vi "magTerm.vi"() -> ()   [LabVIEW 2014]
uses:
  common/crest/LabVIEW/LV14/libcommon-crest.lvlib
panel:
  out "loop":i32
  in  "Simulated/Real":string(combo)
  in  "stop":bool
  out "Array":T1(array[cluster])
  in  "!CHAOS WAN url":string="192.168.150.91:8081"
  in  "Element List":string[](array[string])=["DHSTB001", "DHSTB002", "QUATB001", "QUATB002", "QUATB003", "QUATB004", "QUATB101", "QUATB102"]
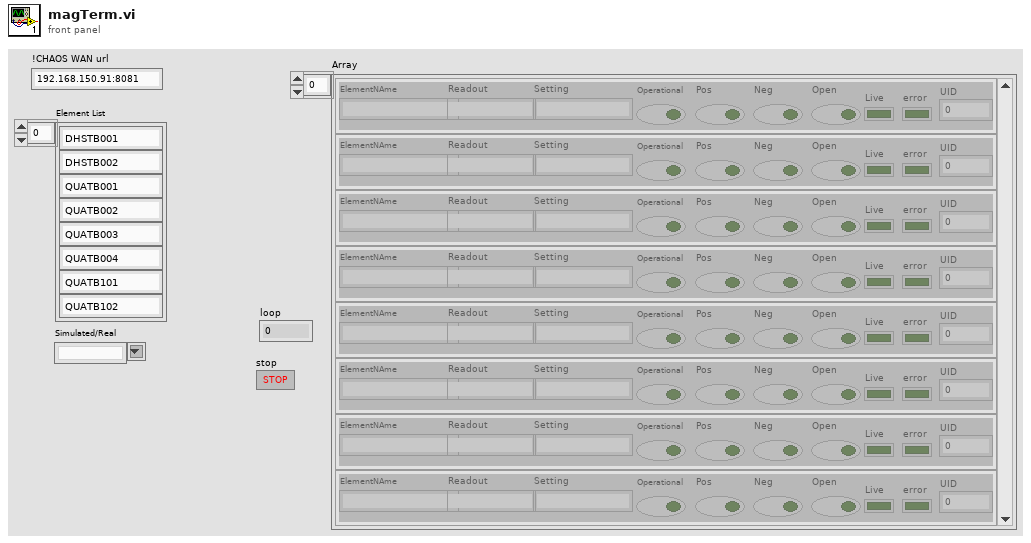
[diagram p1: front panel]
types:
  T1 = cluster{"ElementNAme":string, "Readout":string, "Setting":string, "Operational":bool, "Pos":bool, "Neg ":bool, "Open":bool, "Live":bool, "error":bool, "UID":u32}[]
  T2 = cluster{"ElementNAme":string, "Readout":string, "Setting":string, "Operational":bool, "Pos":bool, "Neg ":bool, "Open":bool, "Live":bool, "error":bool, "UID":u32}
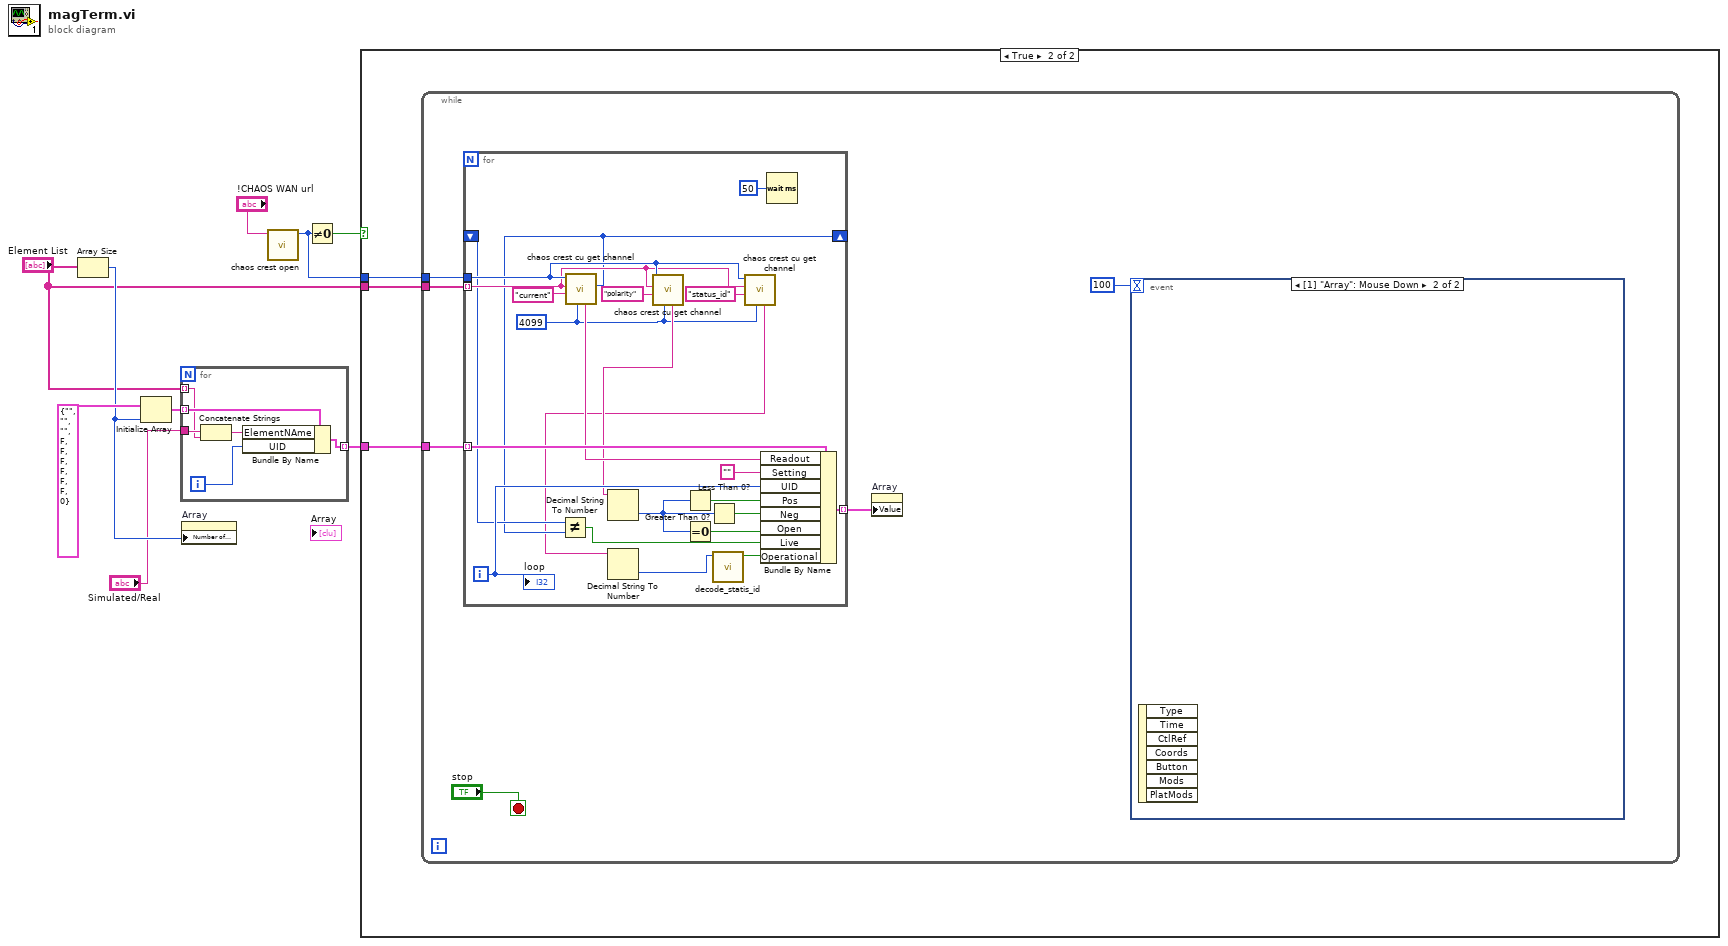
[diagram p0: block diagram]
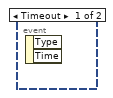
[diagram p3: hidden frame]
diagram:
  n1 = Array Size(array="Element List") -> (size(s)=w6:i32)
  n2 = Initialize Array(T2 {"ElementNAme"="", "Readout"="", "Setting"="", "Operational"=FALSE, "Pos"=FALSE, "Neg "=FALSE, "Open"=FALSE, "Live"=FALSE, "error"=FALSE, "UID"=0} ("magElem"), w6) -> (w8:T1)
  n3 = for {
    tunnel: "Element List" -> [w10] mode=indexing
    tunnel: w8 -> [w15] mode=indexing
    tunnel: [w14] -> w7 mode=indexing
    tunnel: "Simulated/Real" -> [w11]
    i -> [w13]
    n4 = Concatenate Strings(w11, w10) -> (w12:string)
    n5 = Bundle By Name(cluster=w15, "ElementNAme"=w12, "UID"=w13) -> (w14:T2)
  }
  n6 = property on="Array" class="Arr (strict)"("Number of Rows"=w6) -> ()  [unwired: 2 in, 2 out]
  n7 = call "chaos crest open.vi"("chaoswanurl"="!CHAOS WAN url") -> ("function return"=w1:u32)  [unwired: 10 in]
  n8 = Not Equal To 0?(x=w1) -> (x != 0?=w4:bool)
  n9 = case shown="True" w4 {
    tunnel: w7 -> [_ w18]
    tunnel: "Element List" -> [_ w17]
    tunnel: w1 -> [_ w16]
    frame False {
    }
    frame True {
      n10 = while {
        tunnel: w18 -> [w24]
        tunnel: w17 -> [w20]
        tunnel: w16 -> [w19]
        stop <- "stop" stop-if-true
        n11 = for {
          tunnel: w24 -> [w47] mode=indexing
          tunnel: [w43] -> w22 mode=indexing
          tunnel: w20 -> [w33] mode=indexing
          tunnel: w19 -> [w34]
          shift-right: [w30] -> _
          shift-left: _ -> [w31]
          i -> [w44]
          w26 = 4099 ("maxsize")
          n12 = call "chaos crest cu get channel.vi"("maxsize"=w26, "channame"="current", "cuname"=w33, "h"=w34) -> ("timestamp"=w30:u64, "output out"=w45:string)  [unwired: 5 in, 1 out]
          n13 = Not Equal?(x=w31, y=w30) -> (x != y?=w29:bool)
          n14 = call "chaos crest cu get channel.vi"("maxsize"=w26, "channame"="polarity", "cuname"=w33, "h"=w34) -> ("output out"=w39:string)  [unwired: 5 in, 2 out]
          n15 = Decimal String To Number(string=w39) -> (number=w36:i32)  [unwired: 2 in, 1 out]
          n16 = Greater Than 0?(x=w36) -> (x > 0?=w38:bool)
          n17 = Equal To 0?(x=w36) -> (x = 0?=w35:bool)
          n18 = Less Than 0?(x=w36) -> (x < 0?=w37:bool)
          n19 = call "chaos crest cu get channel.vi"("maxsize"=w26, "channame"="status_id", "cuname"=w33, "h"=w34) -> ("output out"=w28:string)  [unwired: 5 in, 2 out]
          n20 = Decimal String To Number(string=w28) -> (number=w27:i32)  [unwired: 2 in, 1 out]
          n21 = call "decode_statis_id.vi"("satatus_id"=w27) -> ("Operational"=w25:bool)  [unwired: 7 in, 3 out]
          n22 = Bundle By Name(cluster=w47, "Readout"=w45, "Setting"="", "UID"=w44, "Pos"=w38, "Neg"=w37, "Open"=w35, "Live"=w29, "Operational"=w25) -> (w43:T2)
          n23 = Wait (ms)(milliseconds to wait=u32 50) -> ()  [unwired: 1 out]
          "loop" <- w44
        }
        n24 = property on="Array" class="Arr (strict)"("Value"=w22) -> ()  [unwired: 2 in, 2 out]
        n25 = event shown="[1] \"Array\": Mouse Down" {
          selector: _ -> [_ _]
          dyn-events: _ -> [_ _]
          timeout: 100 -> [_ _]
          event Timeout {
            n26 = event-data() -> ()  [unwired: 1 in, 2 out]
          }
          event "Array": Mouse Down {
            n27 = event-data() -> ()  [unwired: 1 in, 7 out]
          }
        }
      }
    }
  }
